vi "Chirp_WaitDCV2.vi"(8 "error in (no error)":errorcluster, 11 "ChirpV2 in":refnum<class "ChirpV2.lvclass">) -> (0 "error IO":errorcluster, 1 "data":dynamicdata(graph), 2 "Boolean":bool, 3 "ChirpV2 out":refnum<class "ChirpV2.lvclass">)   [LabVIEW 2014, in "ChirpV2.lvclass"]
uses:
  ChirpV2.lvclass
  <vilib>/measure/NI_MABase.lvlib
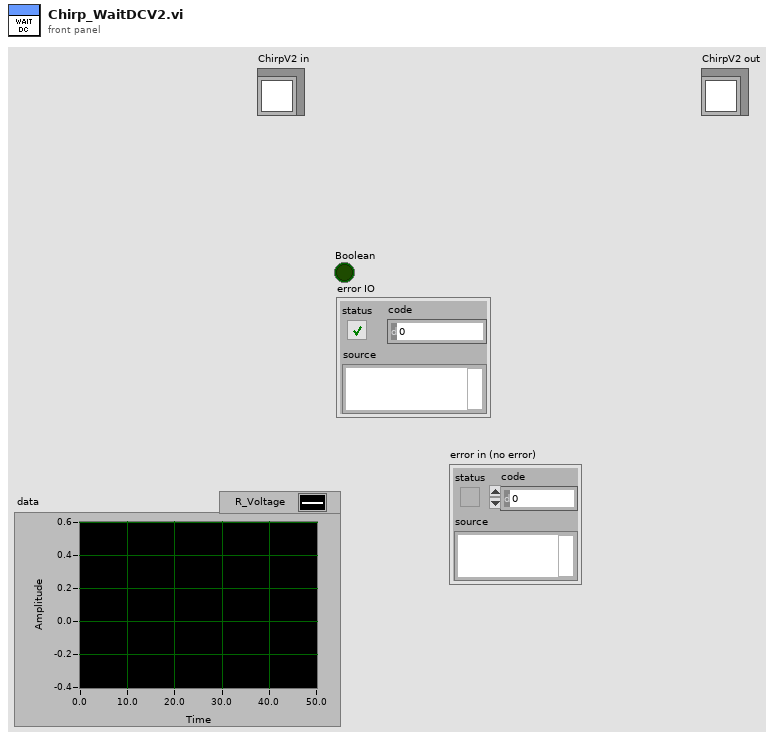
[diagram p1: front panel]
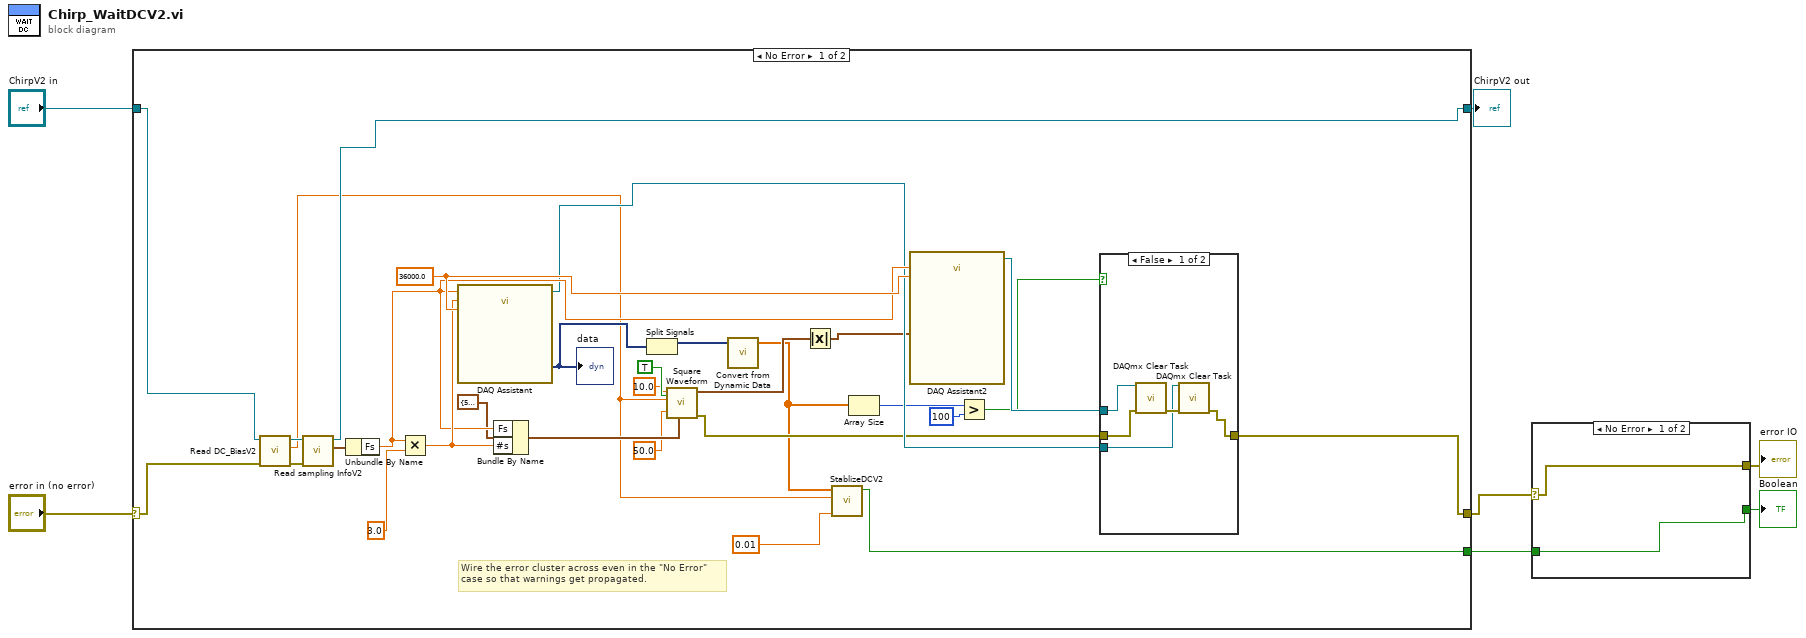
[diagram p0: block diagram]
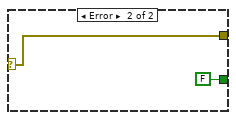
[diagram p2: hidden frame]
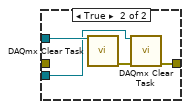
[diagram p3: hidden frame]
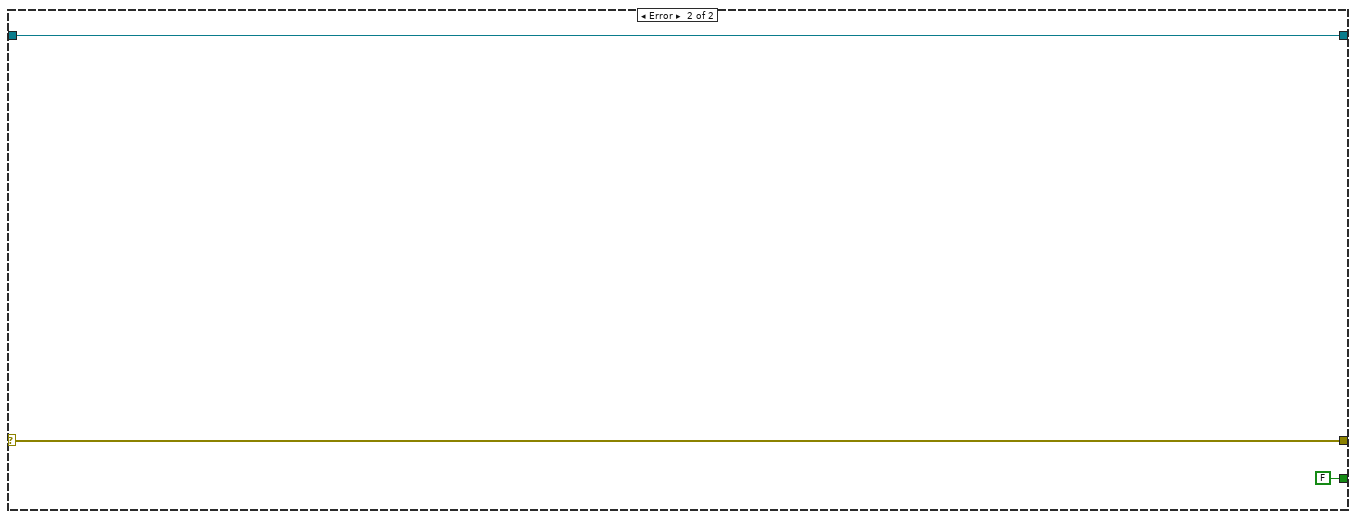
[diagram p4: hidden frame]
diagram:
  n1 = case shown="No Error" "error in (no error)" {
    selector: "error in (no error)" -> [w16 w49]
    tunnel: [w15 w49] -> w4
    tunnel: [w13 w48] -> w5
    tunnel: "ChirpV2 in" -> [w17 w48]
    tunnel: [w8 FALSE ("Boolean")] -> w3
    frame No Error {
      w35 = 36000.0 ("timeout (s)")
      # "Wire the error cluster across even in the \"No Error\"\ncase so that warnings get propagated."
      n2 = call-dynamic "Read DC_BiasV2.vi"("error in (no error)"=w16, "ChirpV2 in"=w17) -> ("error out"=w28:errorcluster, "DC_Bias"=w10:dbl, "ChirpV2 out"=w27:refnum<class "ChirpV2.lvclass">)  [unwired: 7 in]
      n3 = call-dynamic "Read sampling InfoV2.vi"("error in (no error)"=w28, "ChirpV2 in"=w27) -> ("sampling Info"=w29:cluster{"Fs":dbl}, "ChirpV2 out"=w13:refnum<class "ChirpV2.lvclass">)  [unwired: 7 in, 1 out]
      n4 = Unbundle By Name(w29) -> ("Fs"=w33:dbl)
      n5 = Multiply(x=w33, y=3.0) -> (x*y=w34:dbl)
      n6 = call "DAQ Assistant"("rate"=w33, "number of samples"=w34, "timeout (s)"=w35) -> ("task out"=w21:refnum<k21>, "data"=w37:dynamicdata)  [unwired: 14 in, 1 out]
      "data" <- w37
      n7 = Bundle By Name(cluster=cluster{"Fs":dbl, "#s":u32} {"Fs"=51200.0, "#s"=1024} ("sampling info"), "Fs"=w33, "#s"=w34) -> (w31:cluster{"Fs":dbl, "#s":u32})
      n8 = Split Signals(w37) -> (w36:dynamicdata)  [unwired: 2 in, 1 out]
      n9 = call <vilib>:"Square Waveform.vi"("duty cycle (%)"=50.0, "sampling info"=w31, "reset signal"=TRUE, "amplitude"=w10, "frequency"=10.0) -> ("error out"=w12:errorcluster, "signal out"=w25:waveform(dbl))  [unwired: 5 in]
      n10 = call "Convert from Dynamic Data"("Dynamic Data Type"=w36) -> ("Array"=w11:dbl[])  [unwired: 3 in]
      n11 = Absolute Value(x=w25) -> (abs(x)=w14:waveform(dbl))
      n12 = call "StablizeDCV2.vi"("Stability Criteria"=0.01 ("amplitude"), "DC"=w10, "ArrayIn"=w11) -> ("Boolean"=w8:bool)  [unwired: 8 in]
      n13 = Array Size(array=w11) -> (size(s)=w20:i32)
      n14 = call "DAQ Assistant2"("data"=w14, "rate"=w33, "timeout (s)"=w35) -> ("task out"=w22:refnum<k21>)  [unwired: 14 in, 2 out]
      n15 = Greater?(x=w20, y=100) -> (0:w19:bool)
      n16 = case shown="False" w19 {
        tunnel: w21 -> [w40 w45]
        tunnel: w22 -> [w41 w46]
        tunnel: [w38 w43] -> w15
        tunnel: w12 -> [w39 _]
        frame False {
          n17 = call <vilib>:"DAQmx Clear Task.vi"("task in"=w41, "error in"=w39) -> ("error out"=w42:errorcluster)  [unwired: 13 in]
          n18 = call <vilib>:"DAQmx Clear Task.vi"("task in"=w40, "error in"=w42) -> ("error out"=w38:errorcluster)  [unwired: 13 in]
        }
        frame True {
          n19 = call <vilib>:"DAQmx Clear Task.vi"("task in"=w46) -> ("error out"=w44:errorcluster)  [unwired: 14 in]
          n20 = call <vilib>:"DAQmx Clear Task.vi"("task in"=w45, "error in"=w44) -> ("error out"=w43:errorcluster)  [unwired: 13 in]
        }
      }
    }
    frame Error {
    }
  }
  "ChirpV2 out" <- w5
  n21 = case shown="No Error" w4 {
    selector: w4 -> [w50 w52]
    tunnel: w3 -> [w51 _]
    tunnel: [w51 FALSE ("Boolean")] -> w2
    tunnel: [w50 w52] -> w1
    frame No Error {
    }
    frame Error {
    }
  }
  "Boolean" <- w2
  "error IO" <- w1
